vi "Hardware - Setup Analog Input Task and Route Trigger.vi"(4 "error in":errorcluster, 6 "SampClk.Timebase.Src":tag="/Dev3/10MHzRefClock", 7 "task/channels in":refnum<k21>) -> (0 "error out":errorcluster, 2 "SampClk.TimebaseDiv":u32, 3 "task out":refnum<k21>)   [LabVIEW 2009, in "Core SubVIs.lvlib"]
doc: "This VI takes a task configured in Measurement and Automation Explorer (Continuous Analog Acquisition) and sets the timebase to the 10 MHz PXI Clock and routes the start trigger to PXI Trigger Line 0."
uses:
  Core SubVIs.lvlib
  <vilib>/DAQmx/configure/events/hardwareSignals.llb/DAQmx Export Signal (Most Signals).vi
  C:/Program Files/National Instruments/LabVIEW 2009/resource/objmgr/daqmx.rc
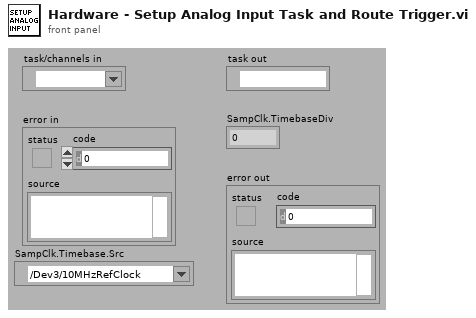
[diagram p1: front panel]
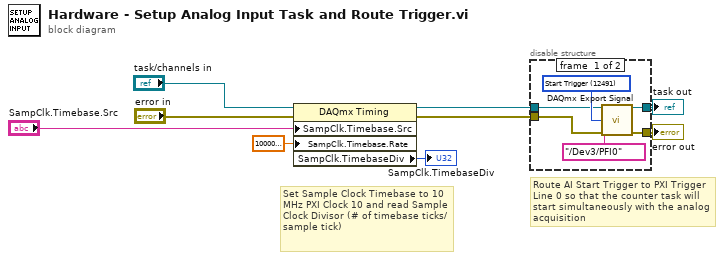
[diagram p0: block diagram]
diagram:
  # "Route AI Start Trigger to PXI Trigger Line 0 so that the counter task will start simultaneously with the analog acquisition"
  # "Set Sample Clock Timebase to 10 MHz PXI Clock 10 and read Sample Clock Divisor (# of timebase ticks/sample tick)"
  n1 = property class="DAQmx Timing"(reference="task/channels in", error in="error in", "SampClk.Timebase.Src"="SampClk.Timebase.Src", "SampClk.Timebase.Rate"=10000000.0) -> (reference out=w2:refnum<k21>, error out=w1:errorcluster, "SampClk.TimebaseDiv"=→"SampClk.TimebaseDiv":u32)
  n2 = disable-structure shown="Enabled" {
    disable-tunnel: [w15 w16] -> w9
    disable-tunnel: [w14 w17] -> w8
    disable-tunnel: w2 -> [w11 w17]
    disable-tunnel: w1 -> [w10 w16]
    frame #0 {
      w13 = 12491 items=["AI Convert Clock"=12484, "10MHz Reference Clock"=12536, "20MHz Timebase Clock"=12486, "Sample Clock"=12487, "Advance Trigger"=12488, "Reference Trigger"=12490, "Start Trigger"=12491, "Advance Complete Event"=12492, "AI Hold Complete Event"=12493, "Counter Output Event"=12494, "Change Detection Event"=12511, "Watchdog Timer Expired Event"=12512] ("signal")
      n3 = call-poly <vilib>:"DAQmx Export Signal.vi"("task/channels in"=w11, "signal"=w13, "output terminal"=tag "/Dev3/PFI0", "error in"=w10) -> ("task out"=w14:refnum<k21>, "error out"=w15:errorcluster)  [unwired: 10 in]
    }
    frame #1 {
    }
  }
  "error out" <- w9
  "task out" <- w8
